vi "2 Wind Records.vi"() -> ()   [LabVIEW 2011]
doc: "This VI is used by the Runprotection VI.\nSTEP 1:\nIt is evaluating the heading of the boat in comparison to the Absolute wind direction, and sets a Warning-Boolean if thos two Values get close (within a certain range).\nSTEP 2:\nIf the Warning is not active, the current wind speed and direction are logged into a global array called WindRecords. This array has a maximum size of 50. \nSTEP 2, cont'd:\nIf warning is active, the Runprotection VI is called."
uses:
  2 Typedefs/absolute wind direction.ctl
  2 Globals/2 Global.vi
panel:
  in  "Run Range":i32=15
  # "This Value is the angle in degrees from the boat to the wind,\nin which the boat counts as running."
  # "This Value sets a range, in which the VI is convinced that it is the actual wind instead of \nrandom occuring values due to running."
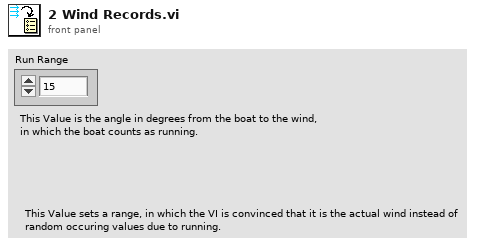
[diagram p1: front panel]
types:
  T1 = typedef "absolute wind direction.ctl" = dbl
  T2 = typedef "absolute wind speed.ctl" = dbl
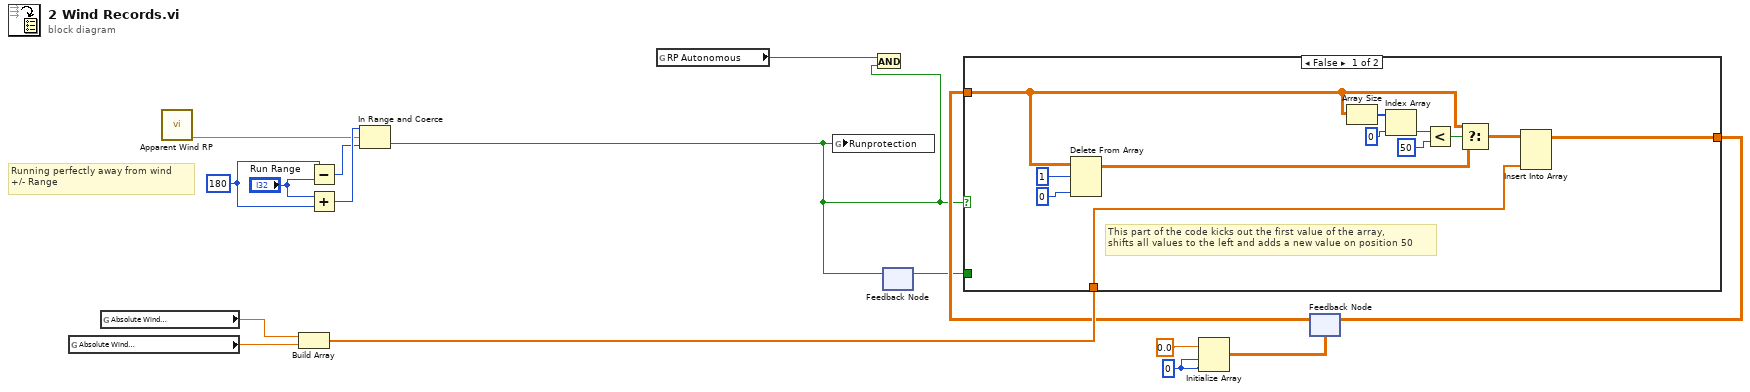
[diagram p0: block diagram]
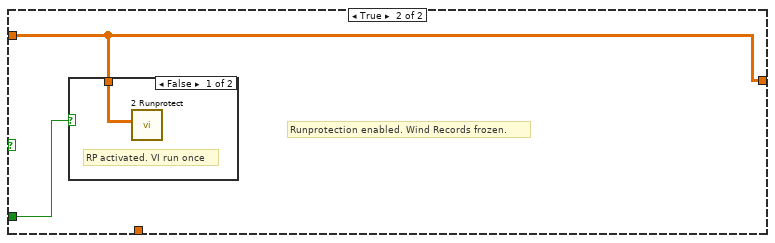
[diagram p2: hidden frame]
diagram:
  w6 = 180
  w9 = 0
  # "Running perfectly away from wind\n+/- Range"
  n1 = global read "2 Global.vi" "Absolute Wind\nDirection (º)"() -> (w15:T1)
  n2 = global read "2 Global.vi" "Absolute Wind\nSpeed"() -> (w16:T2)
  n3 = call "Apparent Wind RP.vi"() -> ("Apparent Wind Direction RP"=w3:dbl)  [unwired: 8 in, 3 out]
  n4 = Build Array(w16, w15) -> (w14:T1[])
  n5 = Subtract(x=w6, y="Run Range") -> (x-y=w4:i32)
  n6 = Add(x="Run Range", y=w6) -> (x+y=w5:i32)
  n7 = In Range and Coerce(upper limit=w5, x=w3, lower limit=w4) -> (In Range?=w1:bool)  [unwired: 1 out]
  n8 = global read "2 Global.vi" "RP Autonomous"() -> (w2:bool)
  n9 = global write "2 Global.vi" "Runprotection"(w1) -> ()
  n10 = And(x=w2, y=w1) -> ()  [unwired: 1 out]
  n11 = feedback #1() -> (w8:bool)  [unwired: 1 in]
  n12 = feedback-in #1(w1) -> ()
  n13 = Initialize Array(T1 0.0 ("Absolute Wind\nDirection (º)"), w9, w9) -> (w10:T1[][])
  n14 = feedback #2(w10) -> (w12:T1[][])
  n15 = case shown="False" w1 {
    tunnel: w14 -> [w28 _]
    tunnel: [w21 w30] -> w13
    tunnel: w12 -> [w20 w30]
    tunnel: w8 -> [_ w29]
    frame False {
      # "This part of the code kicks out the first value of the array, \nshifts all values to the left and adds a new value on position 50"
      n16 = Delete From Array(array=w20, length=1, index (col)=0) -> (array with subset deleted=w17:T1[][])  [unwired: 1 in, 1 out]
      n17 = Array Size(array=w20) -> (size(s)=w27:i32[])
      n18 = Index Array(array=w27, index=0) -> (element=w25:i32)
      n19 = Less?(x=w25, y=50) -> (x < y?=w23:bool)
      n20 = Select(t=w20, s=w23, f=w17) -> (s? t:f=w22:T1[][])
      n21 = Insert Into Array(array=w22, new element=w28) -> (w21:T1[][])  [unwired: 2 in]
    }
    frame True {
      # "Runprotection enabled. Wind Records frozen."
      n22 = case shown="False" w29 {
        tunnel: w30 -> [w31 _]
        frame False {
          # "RP activated. VI run once"
          n23 = call "2 Runprotect.vi"("Wind Records"=w31) -> ()  [unwired: 11 in]
        }
        frame True {
          # "Dont run it all the time"
        }
      }
    }
  }
  n24 = feedback-in #2(w13) -> ()
